vi "Go To Listening.vi"() -> ()   [LabVIEW 2013, in "Receiver.lvlib" / "Receive Commands Using State Actors.lvlib" / "Connect Command.lvlib" / "Connect Command.lvclass"]
uses:
  Connect Command.lvclass
  <vilib>/ni/Actors/State Actor/State Actor/State Actor.lvclass
  States/Listening/Listening.lvclass
panel:
  out "State out":refnum<class "State Actor.lvclass">
  out "error out":errorcluster
  in  "error in (no error)":errorcluster
  in  "Receiver.lvlib:Connect Command.lvlib:Connect Command.lvclass":refnum<class "Connect Command.lvclass">
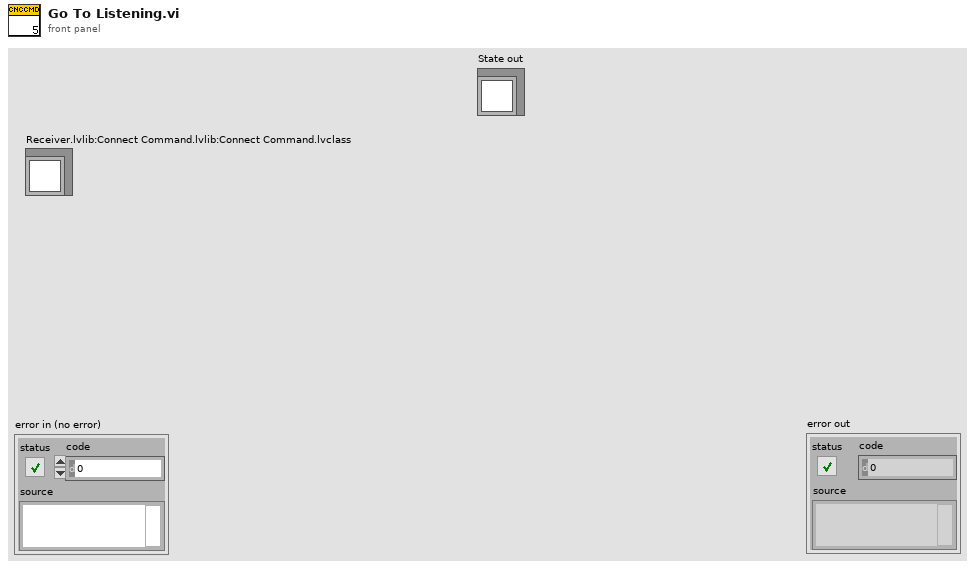
[diagram p1: front panel]
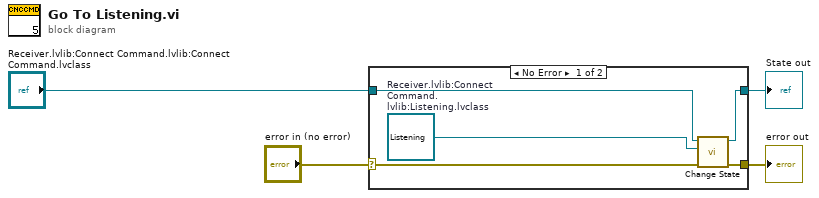
[diagram p0: block diagram]
diagram:
  n1 = case shown="No Error" "error in (no error)" {
    selector: "error in (no error)" -> [w9 w11]
    tunnel: [w8 w11] -> w3
    tunnel: "Receiver.lvlib:Connect Command.lvlib:Connect Command.lvclass" -> [w7 w10]
    tunnel: [w6 w10] -> w1
    frame No Error {
      w5 = refnum<class "Listening.lvclass"> refnum  # Receiver.lvlib:Connect Command.lvlib:Listening.lvclass
      n2 = call <vilib>:"Change State.vi"("error in (no error)"=w9, "New State in"=w5, "State in"=w7) -> ("error out"=w8:errorcluster, "State out"=w6:refnum<class "State Actor.lvclass">)  [unwired: 7 in]
    }
    frame Error {
    }
  }
  "error out" <- w3
  "State out" <- w1
